vi "Read from Property Bag.vi"(8 "error in (no error)":errorcluster, 9 "Data in":variant, 11 "CI Serializer in":refnum<class "CI Serializer.lvclass">) -> (0 "error out":errorcluster, 3 "CI Serializer out":refnum<class "CI Serializer.lvclass">)   [LabVIEW 2014, in "CI Serializer.lvclass"]
uses:
  CI Serializer.lvclass
  CI Serializer.lvclass/CI Serializer.ctl
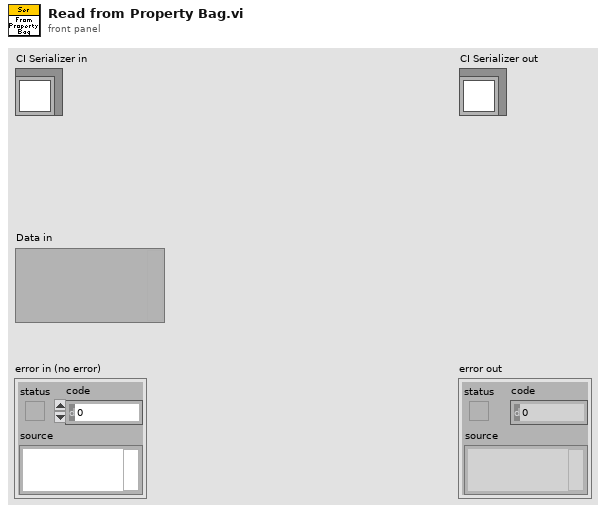
[diagram p1: front panel]
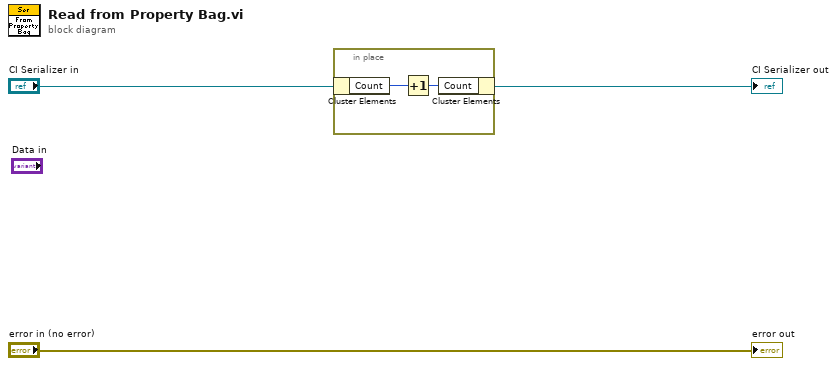
[diagram p0: block diagram]
diagram:
  n1 = in-place {
    n2 = in-place-cluster #1("CI Serializer in") -> ("Count"=w4:i32)
    n3 = Increment(x=w4) -> (x+1=w5:i32)
    n4 = in-place-cluster #1("Count"=w5) -> (→"CI Serializer out":refnum<class "CI Serializer.lvclass">)
  }
  "error out" <- "error in (no error)"
